vi "Channel selection.vi"() -> (0 "channel":u16)   [LabVIEW 2017]
panel:
  in  "정지":bool
  in  "Choose channel to import":u16(slide)
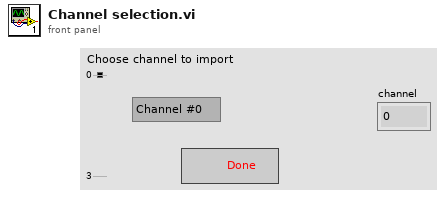
[diagram p1: front panel]
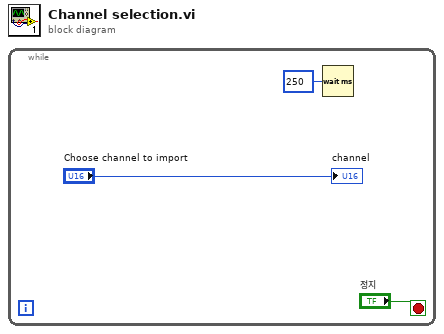
[diagram p0: block diagram]
diagram:
  n1 = while {
    stop <- "정지" stop-if-true
    n2 = Wait (ms)(milliseconds to wait=u32 250 ("대기 시간 (ms)")) -> ()  [unwired: 1 out]
    "channel" <- "Choose channel to import"
  }
